vi "SeCrTs-AO_Write.vi"(7 "Data FIFO Ref":T1, 8 "error in (no error)":errorcluster, 10 "AO_Task":refnum<k21>) -> (0 "error out":errorcluster, 2 "task out":refnum<k21>)   [LabVIEW 2022 SP3]
uses:
  <vilib>/DAQmx/write.llb/DAQmx Write (Analog DBL 1Chan 1Samp).vi
  <vilib>/Platform/TimedLoop/XDataNode/wakeup.ctl
  <vilib>/Platform/TimedLoop/XDataNode/XDNodeRunTimeDep.lvlib
  <vilib>/Platform/TimedLoop/XDataNode/nitl_modes.ctl
  <vilib>/Platform/TimedLoop/XDataNode/timing_clust.ctl
  <vilib>/platform/TimedLoop/XDataNode/XDataNode.xnode
  RT Controls/ATF Storage Haelth.ctl
  RT Controls/SeCrTs-Data FIFO.ctl
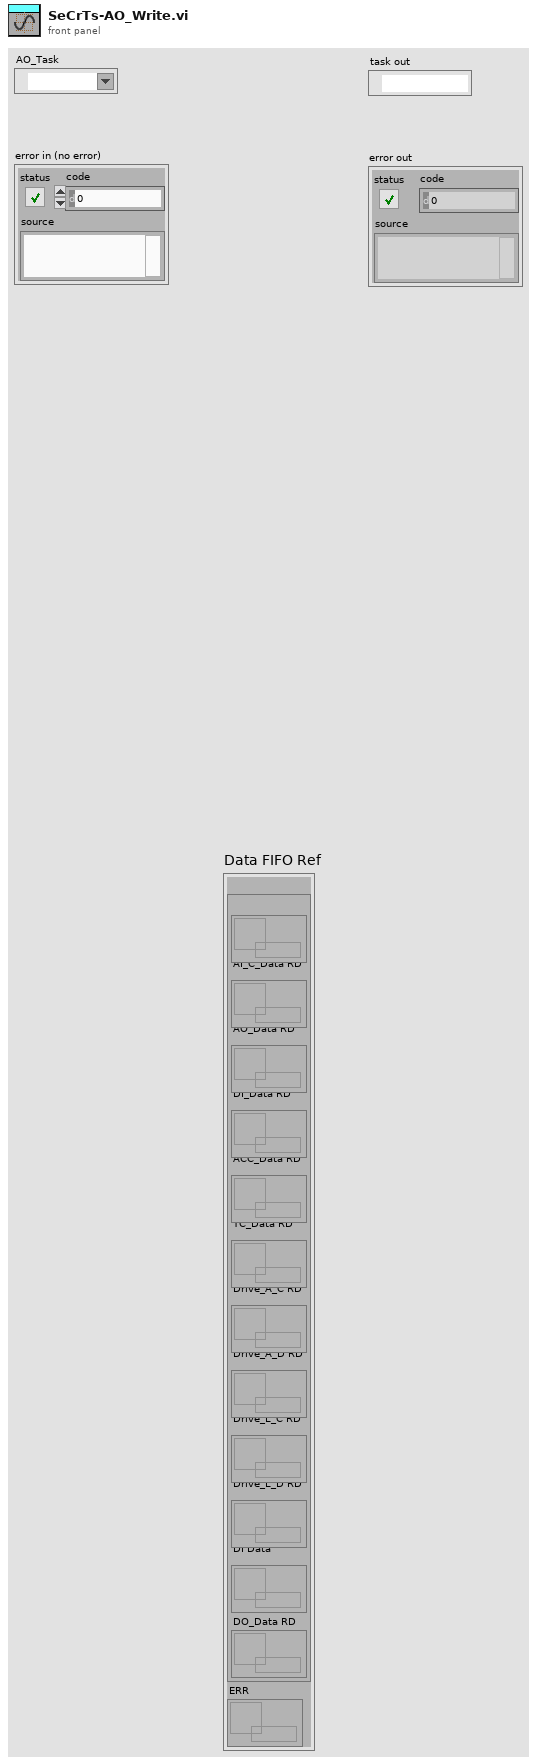
[diagram p1: front panel]
types:
  T1 = typedef "SeCrTs-Data FIFO.ctl" = cluster{"RD":cluster{"AI_V_Data RD":refnum<queue>, "AI_C_Data RD":refnum<queue>, "AO_Data RD":refnum<queue>, "DI_Data RD":refnum<queue>, "ACC_Data RD":refnum<queue>, "TC_Data RD":refnum<queue>, "Drive_A_C RD":refnum<queue>, "Drive_A_D RD":refnum<queue>, "Drive_L_C RD":refnum<queue>, "Drive_L_D RD":refnum<queue>, "DI Data":refnum<queue>, "DO_Data RD":refnum<queue>}, "ERR":refnum<queue>}
  T2 = typedef "XDNodeRunTimeDep.lvlib/timing_clust.ctl" = cluster{"Expected End [f-1]":u64, "Actual End [f-1]":u64, "Finished Late? [f-1]":bool, "Expected End [i-1]":u64, "Actual End [i-1]":u64, "Finished Late? [i-1]":bool, "Expected Start [i]":u64, "Actual Start [i]":u64, "Expected Start [f]":u64, "Actual Start [f]":u64, "Source Name":string, "Structure Name":string, "Period":i64, "Deadline":i64, "Offset":i64, "Start":i64, "Priority":i32, "Timeout":i32, "Mode":T3, "Wakeup Reason":T4, "Error":errorcluster, "Source Type":string, "Secondary Source Type":string, "Global End Time":u64, "Global Start Time":u64, "Frame Duration":u64, "Iteration Duration":u64, "Assigned CPU":i32, "I/O Scan Engine Mode":u32}
  T3 = typedef "XDNodeRunTimeDep.lvlib/nitl_modes.ctl" = enum32{"No Change", "Process missed periods, maintain original phase", "Discard missed periods, maintain original phase", "Process missed periods, ignore original phase", "Discard missed periods, ignore original phase"}
  T4 = typedef "XDNodeRunTimeDep.lvlib/wakeup.ctl" = enum32{"Normal", "Aborted", "Asynchronous wakeup", "Timing source error", "Timed loop error", "Timeout"}
  T5 = typedef "ATF Storage Haelth.ctl" = enum16{"AI C", "AI V", "AO", "DI", "DO", "TC", "ACC", "RT Str", "DR A"}
  T6 = enum16{"Init", "Read 'All'", "Read 'n'", "Read '1'", "Write '1'", "Write 'n'", "Write 'All'"}
  T7 = cluster{"Start DAQ":bool, "Stop DAQ":bool, "RT Stop":bool, "RT Exit":bool, "Start Seq":bool}
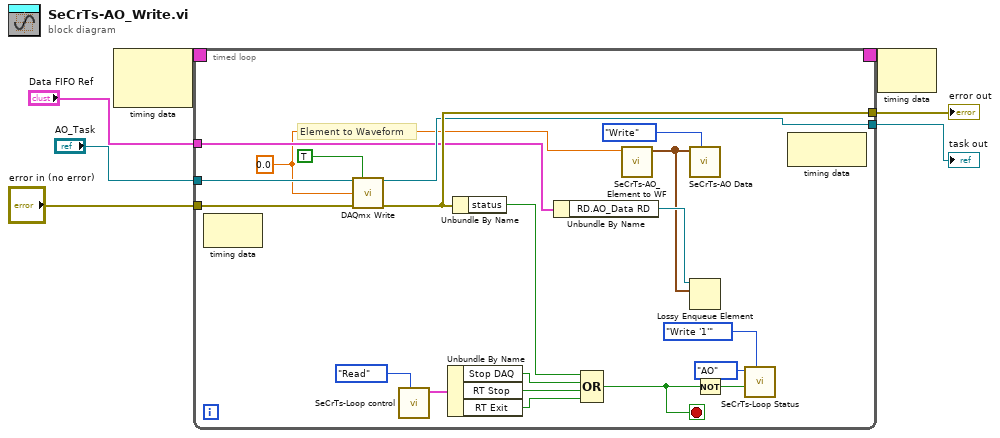
[diagram p0: block diagram]
diagram:
  n1 = node-c288() -> (w7:T2)  [unwired: 2 in]
  n2 = timed-loop {
    tunnel: [w27] -> w2
    tunnel: "AO_Task" -> [w25]
    tunnel: "error in (no error)" -> [w24]
    tunnel: [w21] -> w5
    timing: w7 -> [_]
    timing-out: [_] -> w6
    tunnel: "Data FIFO Ref" -> [w14]
    stop <- w22 stop-if-true
    w11 = 0.0 ("data")
    # "Element to Waveform"
    n3 = node-c288() -> ()  [unwired: 1 in, 1 out]
    n4 = call-poly <vilib>:"DAQmx Write.vi"("task/channels in"=w25, "auto start"=TRUE, "data"=w11, "error in"=w24) -> ("task out"=w21:refnum<k21>, "error out"=w27:errorcluster)  [unwired: 9 in, 1 out]
    n5 = call "SeCrTs-Loop control.vi"("Action"=enum16{"Init", "Write", "Read"}."Read") -> ("Loop Control out"=w19:T7)  [unwired: 9 in, 1 out]
    n6 = Unbundle By Name(w19) -> ("Stop DAQ"=w18:bool, "RT Stop"=w17:bool, "RT Exit"=w16:bool)
    n7 = Unbundle By Name(w27) -> ("status"=w23:bool)
    n8 = Unbundle By Name(w14) -> ("RD.AO_Data RD"=w13:refnum<queue>)
    n9 = Compound Arithmetic op=OR(w23, w18, w17, w16) -> (w22:bool)
    n10 = call "SeCrTs-AO_Element to WF.vi"("AO Array"=w11) -> ("Array"=w12:waveform(dbl)[])  [unwired: 10 in]
    n11 = call "SeCrTs-AO Data.vi"("Enum"=enum16{"Write", "Read"}."Write", "In_DO data"=w12) -> ()  [unwired: 9 in, 1 out]
    n12 = Lossy Enqueue Element(queue=w13, element=w12) -> ()  [unwired: 1 in, 4 out]
    n13 = Not(x=w22) -> (.not. x?=w9:bool)
    n14 = call "SeCrTs-Loop Status.vi"("Option"=T6."Write '1'", "Status"=w9, "Loop"=ATF_Storage_Haelth."AO") -> ()  [unwired: 6 in, 3 out]
    n15 = node-c288() -> ()  [unwired: 1 in, 1 out]
  }
  "task out" <- w5
  "error out" <- w2
  n16 = node-c288(w6) -> ()  [unwired: 1 out]
